vi "Migrate all Measurement Dependencies.vi"(0 "Project path":path, 1 "Measurement paths":path[](array[path]), 5 "Plug-in names":string[](array[string]), 7 "Measurement dependencies":path[][](array[path]), 9 "Outside items":string[](array[string]), 11 "error in (no error)":errorcluster, 12 "Shared dependent VIs":path[](array[path])) -> (15 "error out":errorcluster)   [LabVIEW 2021]
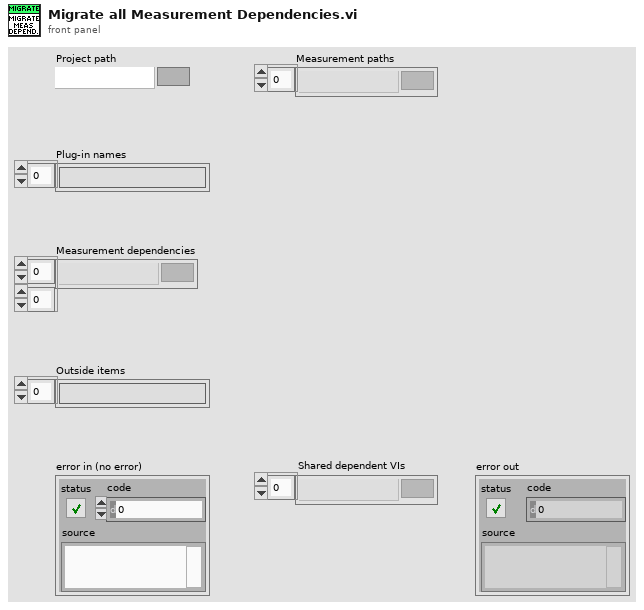
[diagram p1: front panel]
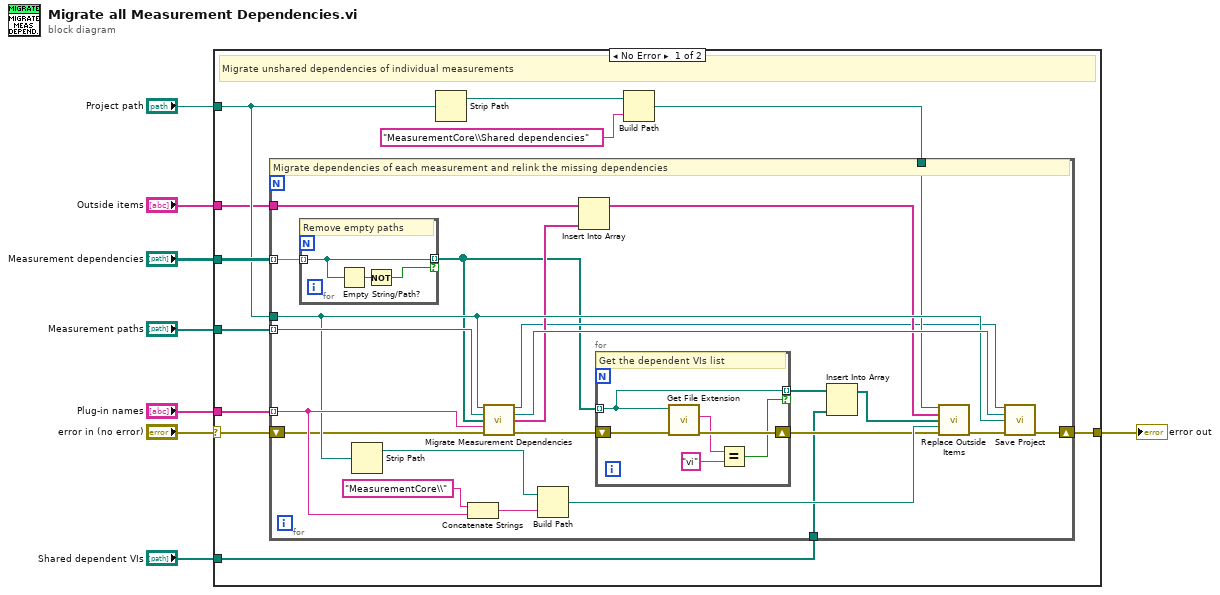
[diagram p0: block diagram]
diagram:
  n1 = case shown="No Error" "error in (no error)" {
    selector: "error in (no error)" -> [w18 w52]
    tunnel: "Measurement dependencies" -> [w19 _]
    tunnel: "Project path" -> [w14 _]
    tunnel: "Outside items" -> [w13 _]
    tunnel: "Measurement paths" -> [w12 _]
    tunnel: "Plug-in names" -> [w11 _]
    tunnel: [w10 w52] -> w2
    tunnel: "Shared dependent VIs" -> [w9 _]
    frame No Error {
      # "Migrate unshared dependencies of individual measurements"
      n2 = Strip Path(path=w14) -> (stripped path=w15:path)  [unwired: 1 out]
      n3 = Build Path(base path=w15, name or relative path="MeasurementCore\\Shared dependencies" ("string")) -> (appended path=w17:path)
      n4 = for {
        tunnel: w14 -> [w34]
        tunnel: w12 -> [w39] mode=indexing
        tunnel: w11 -> [w36] mode=indexing
        tunnel: w13 -> [w33]
        tunnel: w17 -> [w29]
        shift-right: [w40] -> w10
        shift-left: w18 -> [w27]
        tunnel: w19 -> [w26] mode=indexing
        tunnel: w9 -> [w21]
        # "Migrate dependencies of each measurement and relink the missing dependencies"
        n5 = for {
          tunnel: w26 -> [w50] mode=indexing
          tunnel: [w50] -> w23 mode=indexing if=w49
          # "Remove empty paths"
          n6 = Empty String/Path?(string/path=w50) -> (empty?=w51:bool)
          n7 = Not(x=w51) -> (.not. x?=w49:bool)
        }
        n8 = Strip Path(path=w34) -> (stripped path=w35:path)  [unwired: 1 out]
        n9 = Concatenate Strings("MeasurementCore\\" ("string"), w36) -> (w24:string)
        n10 = call "Migrate Measurement Dependencies.vi"("Project path"=w34, "Measurement path"=w39, "Dependencies path"=w23, "Plug-in name"=w36, "error in (no error)"=w27) -> ("Project reference"=w28:refnum<vi>, "MeasurementCore reference"=w38:refnum<vi>, "Outside items"=w32:string[], "error out"=w42:errorcluster)  [unwired: 7 in]
        n11 = Build Path(base path=w35, name or relative path=w24) -> (appended path=w30:path)
        n12 = Insert Into Array(array=w33, new element=w32) -> (w31:string[])  [unwired: 1 in]
        n13 = for {
          shift-right: [w47] -> w25
          shift-left: w42 -> [w48]
          tunnel: w23 -> [w46] mode=indexing
          tunnel: [w46] -> w22 mode=indexing if=w43
          # "Get the dependent VIs list"
          n14 = call <vilib>:"Get File Extension.vi"("error in (no error)"=w48, "file"=w46) -> ("error out"=w47:errorcluster, "lowercase file extension"=w44:string)  [unwired: 5 in, 3 out]
          n15 = Equal?(x=w44, y="vi" ("x")) -> (x = y?=w43:bool)
        }
        n16 = Insert Into Array(array=w22, new element=w21) -> (w20:path[])  [unwired: 1 in]
        n17 = call "Replace Outside Items.vi"("Shared directory"=w29, "OutsideVIs"=w31, "Dependent VIs"=w20, "Measurement directory"=w30, "error in (no error)"=w25) -> ("error out"=w41:errorcluster)  [unwired: 10 in]
        n18 = call "Save Project.vi"("Project reference"=w28, "MeasurementCore reference"=w38, "Project path"=w34, "error in (no error)"=w41) -> ("error out"=w40:errorcluster)  [unwired: 11 in]
      }
    }
    frame Error {
      # "Pass"
    }
  }
  "error out" <- w2
